vi "식노드.vi"() -> ()   [LabVIEW 2014]
panel:
  out "N 2":dbl format="%#_16f"
  in  "N":dbl
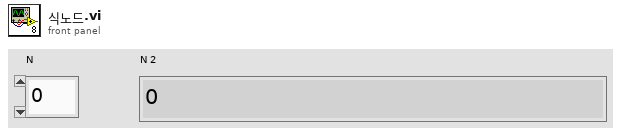
[diagram p1: front panel]
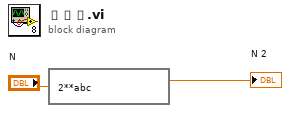
[diagram p0: block diagram]
diagram:
  n1 = expression code="2**abc"("N") -> (→"N 2":dbl)
